vi "Show Front Panel.vi"(4 "Window Vertical Size (pixels)":i16=600, 6 "Window Horizontal Size (pixels)":i16=800, 8 "Error In":errorcluster, 11 "VI Reference":refnum<vi>) -> (0 "Error Out":errorcluster)   [LabVIEW 2023, in "Error Manager.lvlib"]
doc: "This VI configures the front panel window of the Error Manager Main VI. This VI is expected to be called when the user presses the button that enables them to view the list of errors that may have occurred in the application up to that point."
uses:
  Error Manager.lvlib
  <vilib>/Utility/miscctls.llb/LVPointTypeDef.ctl
  <vilib>/Utility/miscctls.llb/LVRectTypeDef.ctl
panel:
  # "Development\ncontrols/indicators useful for development and testing, but which are not outputs of the VI"
  # "Input\nInputs to the VI"
  # "Output\nOutputs of the VI"
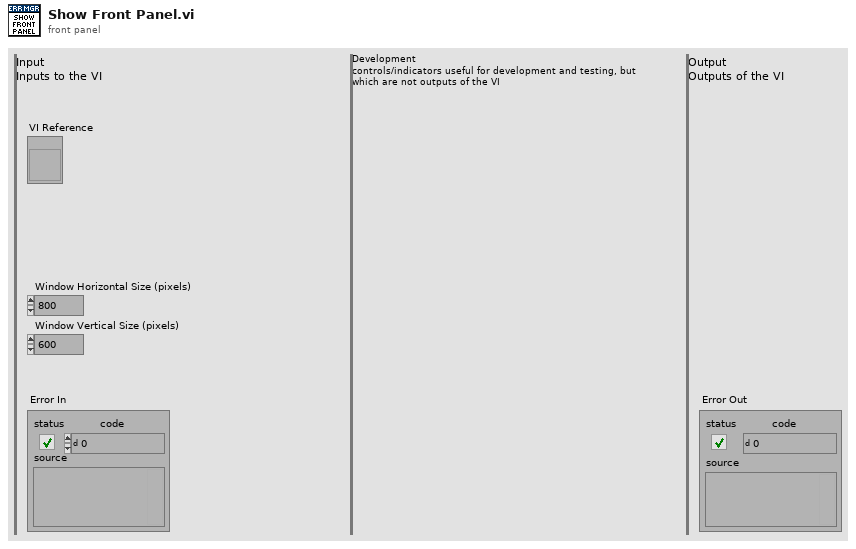
[diagram p1: front panel]
types:
  T1 = enum32{"Invalid", "Standard", "Closed", "Hidden", "Minimized", "Maximized"}
  T2 = enum32{"Invalid", "Default", "Floating", "Floating/Auto-Hide", "Modal"}
  T3 = typedef "LVRectTypeDef.ctl" = cluster{"Left":i16, "Top":i16, "Right":i16, "Bottom":i16}
  T4 = typedef "LVPointTypeDef.ctl" = cluster{"Horizontal":i16, "Vertical":i16}
  T5 = enum16{"Always On", "Always Off", "Off While Running"}
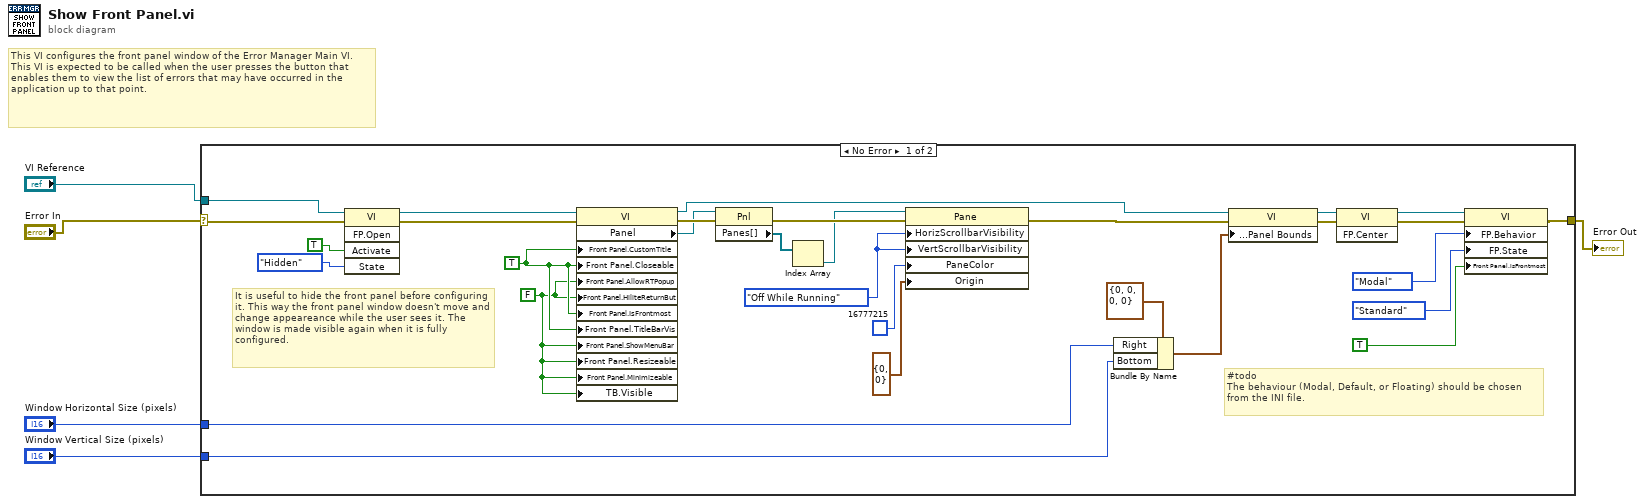
[diagram p0: block diagram]
diagram:
  # "This VI configures the front panel window of the Error Manager Main VI. This VI is expected to be called when the user presses the button that enables them to view the list of errors that may have occurred in the application up to that point."
  n1 = case shown="No Error" "Error In" {
    selector: "Error In" -> [w15 w36]
    tunnel: [w7 w36] -> w3
    tunnel: "VI Reference" -> [w13 _]
    tunnel: "Window Horizontal Size (pixels)" -> [w19 _]
    tunnel: "Window Vertical Size (pixels)" -> [w18 _]
    frame No Error {
      w29 = T5."Off While Running" ("Horizontal Scrollbar Visibility")
      w27 = FALSE
      w34 = TRUE
      # "It is useful to hide the front panel before configuring it. This way the front panel window doesn't move and change appeareance while the user sees it. The window is made visible again when it is fully configured."
      # "#todo\nThe behaviour (Modal, Default, or Floating) should be chosen from the INI file."
      n2 = invoke class="VI" method="FP.Open"(reference=w13, error in=w15, "Activate"=TRUE ("Activate?"), "State"=T1."Hidden") -> (reference out=w12:refnum<vi>, error out=w14:errorcluster)  [unwired: 1 in, 3 out]
      n3 = property class="VI"(reference=w12, error in=w14, "Front Panel.CustomTitle"=w34, "Front Panel.Closeable"=w34, "Front Panel.AllowRTPopup"=w27, "Front Panel.HiliteReturnBut"=w27, "Front Panel.IsFrontmost"=w34, "Front Panel.TitleBarVis"=w34, "Front Panel.ShowMenuBar"=w27, "Front Panel.Resizeable"=w27, "Front Panel.Minimizeable"=w27, "TB.Visible"=w27) -> (reference out=w23:refnum<vi>, error out=w35:errorcluster, "Panel"=w32:refnum<vi>)
      n4 = property class="Pnl"(reference=w32, error in=w35) -> (error out=w33:errorcluster, "Panes[]"=w31:refnum<vi>[])  [unwired: 1 out]
      n5 = Index Array(array=w31) -> (element=w30:refnum<vi>)  [unwired: 1 in]
      n6 = property class="Pane"(reference=w30, error in=w33, "HorizScrollbarVisibility"=w29, "VertScrollbarVisibility"=w29, "PaneColor"=u32 16777215, "Origin"=T4 {"Horizontal"=0, "Vertical"=0}) -> (error out=w25:errorcluster)  [unwired: 1 out]
      n7 = Bundle By Name(cluster=T3 {"Left"=0, "Top"=0, "Right"=0, "Bottom"=0} ("Front Panel Window:Panel Bounds"), "Right"=w19, "Bottom"=w18) -> (w21:T3)
      n8 = property on="Property Node" class="VI"(reference=w23, error in=w25, "Front Panel Window:Panel Bounds"=w21) -> (reference out=w20:refnum<vi>, error out=w24:errorcluster)
      n9 = invoke class="VI" method="FP.Center"(reference=w20, error in=w24) -> (reference out=w6:refnum<vi>, error out=w8:errorcluster)  [unwired: 1 in, 1 out]
      n10 = property class="VI"(reference=w6, error in=w8, "FP.Behavior"=T2."Modal" ("Front Panel Window:Behavior"), "FP.State"=T1."Standard" ("Front Panel Window:State"), "Front Panel.IsFrontmost"=TRUE ("Front Panel Window:Is Frontmost")) -> (error out=w7:errorcluster)  [unwired: 1 out]
    }
    frame Error {
    }
  }
  "Error Out" <- w3
